vi "test - Module Name Case Insensitive.vi"(8 "error in (no error)":errorcluster, 11 "TestCase in":refnum<class "testcase-Basic-Function.lvclass">) -> (0 "error out":errorcluster, 3 "TestCase out":refnum<class "testcase-Basic-Function.lvclass">)   [LabVIEW 2017, in "testcase-Basic-Function.lvclass"]
uses:
  testcase-Basic-Function.lvclass
  <vilib>/addons/_JKI Toolkits/VI Tester/TestCase.llb/TestCase.lvclass
  user.lib/_NEVSTOP/Communicable State Machine(CSM)/Communicable State Machine.lvlib
  C:/Program Files (x86)/National Instruments/LabVIEW 2017/vi.lib/addons/_JKI Toolkits/VI Tester/TestCase.llb/TestCase.lvclass
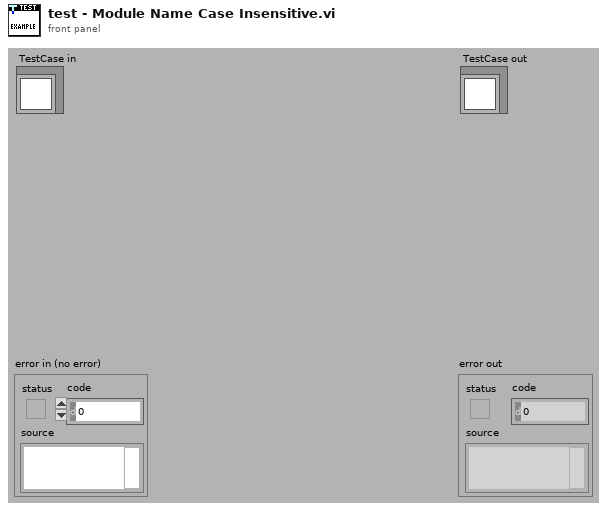
[diagram p1: front panel]
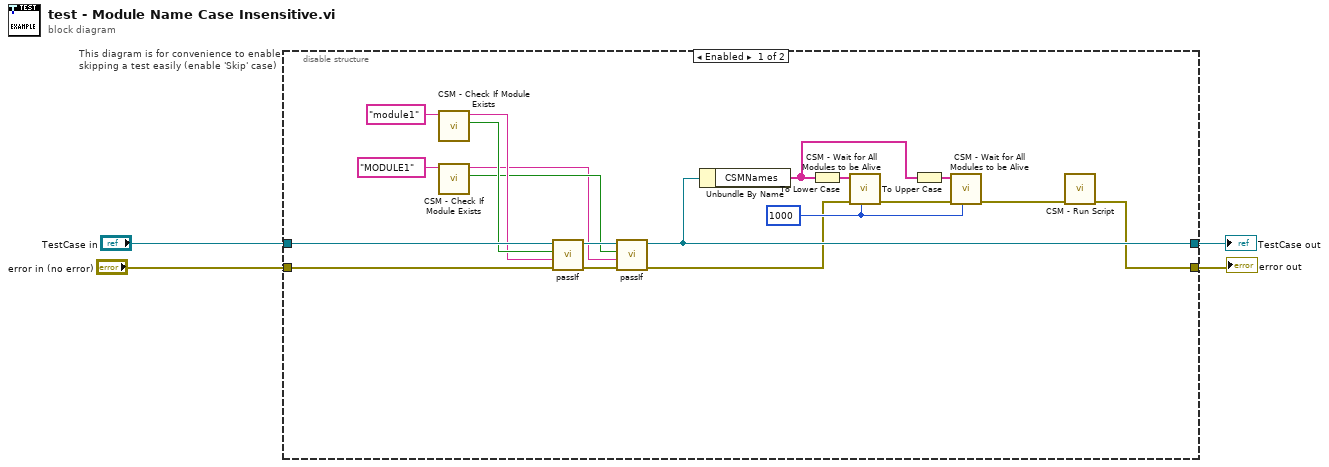
[diagram p0: block diagram]
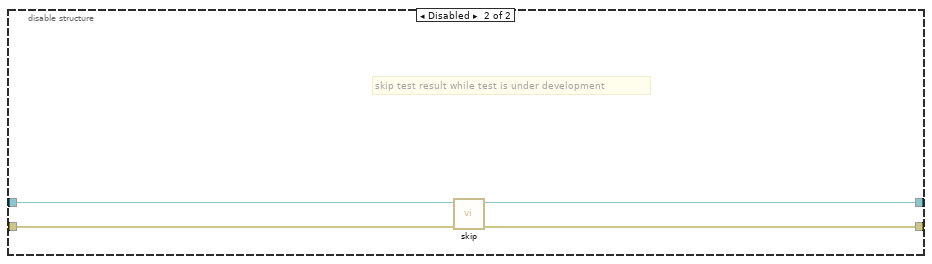
[diagram p2: hidden frame]
diagram:
  n1 = disable-structure "This diagram is for convenience to enable skipping a test easily (enable 'Skip' case)" shown="Enabled" {
    disable-tunnel: "TestCase in" -> [w23 w27]
    disable-tunnel: [w13 w25] -> w1
    disable-tunnel: [w5 w26] -> w3
    disable-tunnel: "error in (no error)" -> [w22 w24]
    frame Enabled {
      w12 = u32 1000 ("Timeout(5000ms)")
      n2 = call "CSM - Check If Module Exists.vi"("CSM Name"="module1") -> ("Exist?"=w19:bool, "CSM Name(dup)"=w18:string)  [unwired: 8 in, 1 out]
      n3 = call "CSM - Check If Module Exists.vi"("CSM Name"="MODULE1") -> ("Exist?"=w15:bool, "CSM Name(dup)"=w14:string)  [unwired: 8 in, 1 out]
      n4 = call-dynamic "passIf.vi"("error in (no error)"=w22, "message (\"\")"=w18, "pass"=w19, "TestCase in"=w23) -> ("error out"=w17:errorcluster, "TestCase out"=w16:refnum<class "testcase-Basic-Function.lvclass">)  [unwired: 6 in]
      n5 = call-dynamic "passIf.vi"("error in (no error)"=w17, "message (\"\")"=w14, "pass"=w15, "TestCase in"=w16) -> ("error out"=w10:errorcluster, "TestCase out"=w13:refnum<class "testcase-Basic-Function.lvclass">)  [unwired: 6 in]
      n6 = Unbundle By Name(w13) -> ("CSMNames"=w11:string[])
      n7 = To Lower Case(string=w11) -> (all lower case string=w7:string[])
      n8 = call "CSM - Wait for All Modules to be Alive.vi"("Timeout(5000ms)"=w12, "Error in"=w10, "Module Names (in)"=w7) -> ("Error out"=w9:errorcluster)  [unwired: 6 in, 2 out]
      n9 = To Upper Case(1:w11) -> (0:w6:string[])
      n10 = call "CSM - Wait for All Modules to be Alive.vi"("Timeout(5000ms)"=w12, "Error in"=w9, "Module Names (in)"=w6) -> ("Error out"=w8:errorcluster)  [unwired: 6 in, 2 out]
      n11 = call "CSM - Run Script.vi"("error in (no error)"=w8) -> ("error out"=w5:errorcluster)  [unwired: 13 in, 1 out]
    }
    frame Disabled {
      # "skip test result while test is under development"
      n12 = call <vilib>:"skip.vi"("error in (no error)"=w24, "TestCase in"=w27) -> ("error out"=w26:errorcluster, "TestCase out"=w25:refnum<class "testcase-Basic-Function.lvclass">)  [unwired: 8 in]
    }
  }
  "error out" <- w3
  "TestCase out" <- w1
